vi "SV TDMS Read Even-Angle Channel Info.vi"(8 "error in":errorcluster, 9 "channel name in":string, 10 "group name in":string, 11 "tdms file":refnum<k34>) -> (0 "error out":errorcluster, 1 "channel name out":string, 2 "group name out":string, 3 "tdms file out":refnum<k34>, 4 "even-angle channel info":T2 {"channel info"."pregain" format="%.2f"; "channel info"."weighting filter" items=["Linear", "A-weighting", "B-weighting", "C-weighting", "ITU-R 468-4", "Dolby", "CCITT", "C-message", "Wb", "Wc", "Wd", "We", "Wf", "Wh", "Wj", "Wk", "Wm", "AES17 20 kHz lowpass", "AES17 40 kHz lowpass", "AES17 20 kHz highpass", "AES17 40 kHz highpass"]; "channel info"."dB reference" format="%^.1e"; "channel info"."engineering units" items=["custom..."=0, "V"=1, "A"=21, "C"=30, "pC"=31, "s"=32, "-"=29, "Pa"=2, "N"=20, "g"=3, "m/s^2"=4, "m/s"=5, "m"=6, "mm/s"=12, "mm"=13, "micron/s"=14, "micron"=15, "in/s^2"=7, "in/s"=8, "in"=9, "mil/s"=10, "mil"=11, "rad/s^2"=16, "rad/s"=17, "rad"=18, "deg/s^2"=26, "deg/s"=27, "deg"=28, "RPM"=22, "cycle/s^2"=23, "Hz"=24, "cycle"=25, "strain"=19]; "channel info"."sensor sensitivity" format="%#_5f"}, 6 "scale labels":T1)   [LabVIEW 2017]
uses:
  <vilib>/addons/_NISVFA/_Shared subVIs/Controls/svc_Resampled Channel Info.ctl
  <vilib>/addons/_NISVFA/_Shared subVIs/Controls/svc_Channel Info.ctl
  <vilib>/addons/_NISVFA/_Shared subVIs/Controls/svc_Engineering Units Text Ring.ctl
  <vilib>/addons/_NISVFA/_Shared subVIs/Controls/svc_Weighting Filter Text Ring.ctl
  <vilib>/addons/_NISVFA/_Shared subVIs/Controls/NI Channel Properties.ctl
  <vilib>/addons/_NISVFA/_Shared subVIs/Controls/SV Channel Properties.ctl
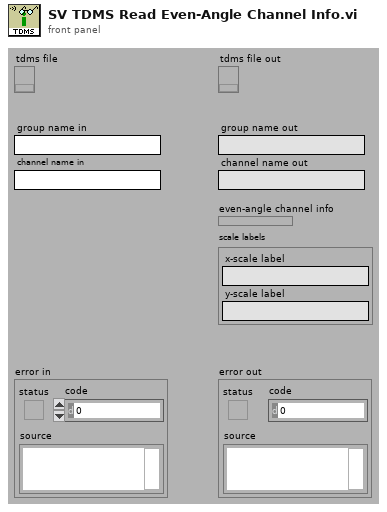
[diagram p1: front panel]
types:
  T1 = cluster{"x-scale label":string, "y-scale label":string}
  T2 = typedef "svc_Resampled Channel Info.ctl" = cluster{"channel name":string, "description":string, " channel info":T3}
  T3 = typedef "svc_Channel Info.ctl" = cluster{"sensor sensitivity":dbl, "engineering units":T4, "dB reference":dbl, "custom label":string, "weighting filter":T5, "pregain":dbl}
  T4 = typedef "svc_Engineering Units Text Ring.ctl" = u16
  T5 = typedef "svc_Weighting Filter Text Ring.ctl" = u16
  T6 = typedef "NI Channel Properties.ctl" = u16
  T7 = typedef "SV Channel Properties.ctl" = u16
  T8 = cluster{"scale label with units":string, "scale label with units":string}
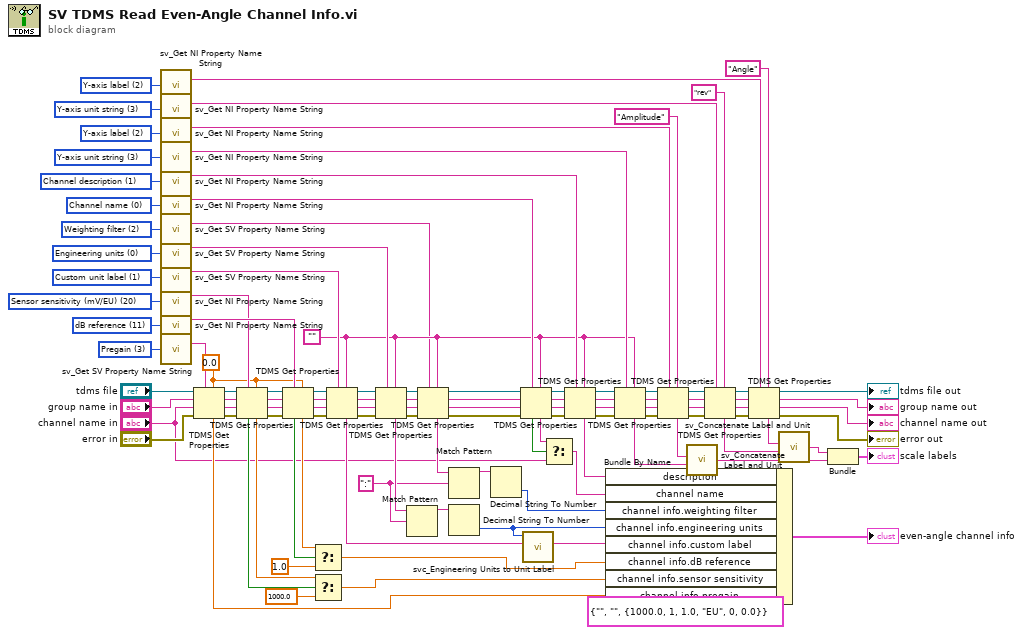
[diagram p0: block diagram]
diagram:
  w28 = T6 2 items=["Channel name", "Channel description", "Y-axis label", "Y-axis unit string", "X-axis label", "X-axis unit string", "x0", "dx", "Number of samples", "X channel", "Filter settled", "dB reference", "Window", "Window parameter", "Window size", "FFT size", "Peak units", "Spectrum type", "Magnitude scale", "Spectral density"] ("property")
  w27 = T6 3 items=["Channel name", "Channel description", "Y-axis label", "Y-axis unit string", "X-axis label", "X-axis unit string", "x0", "dx", "Number of samples", "X channel", "Filter settled", "dB reference", "Window", "Window parameter", "Window size", "FFT size", "Peak units", "Spectrum type", "Magnitude scale", "Spectral density"] ("property")
  w80 = T6 20 items=["Channel name", "Channel description", "Y-axis label", "Y-axis unit string", "X-axis label", "X-axis unit string", "x0", "dx", "Number of samples", "X channel", "Filter settled", "dB reference", "Window", "Window parameter", "Window size", "FFT size", "Peak units", "Spectrum type", "Magnitude scale", "Spectral density", "Sensor sensitivity (mV/EU)", "X-axis domain", "LabVIEW datatype"] ("property")
  w58 = ":" ("regular expression")
  w62 = "" ("channel info.custom label")
  w13 = 0.0 ("property values")
  w71 = T6 0 items=["Channel name", "Channel description", "Y-axis label", "Y-axis unit string", "X-axis label", "X-axis unit string", "x0", "dx", "Number of samples", "X channel", "Filter settled", "dB reference", "Window", "Window parameter", "Window size", "FFT size", "Peak units", "Spectrum type", "Magnitude scale", "Spectral density", "Sensor sensitivity (mV/EU)"] ("property")
  w74 = T6 11 items=["Channel name", "Channel description", "Y-axis label", "Y-axis unit string", "X-axis label", "X-axis unit string", "x0", "dx", "Number of samples", "X channel", "Filter settled", "dB reference", "Window", "Window parameter", "Window size", "FFT size", "Peak units", "Spectrum type", "Magnitude scale", "Spectral density"] ("property")
  w75 = T7 3 items=["Engineering units", "Custom unit label", "Weighting filter", "Pregain", "Octave standard", "Octave bandwidth", "Octave low band", "Octave high band", "Spectrum skewed"] ("SV property")
  w79 = T6 2 items=["Channel name", "Channel description", "Y-axis label", "Y-axis unit string", "X-axis label", "X-axis unit string", "x0", "dx", "Number of samples", "X channel", "Filter settled", "dB reference", "Window", "Window parameter", "Window size", "FFT size", "Peak units", "Spectrum type", "Magnitude scale", "Spectral density"] ("property")
  w81 = T7 1 items=["Engineering units", "Custom unit label", "Weighting filter", "Pregain", "Octave standard", "Octave bandwidth", "Octave low band", "Octave high band", "Spectrum skewed"] ("SV property")
  w82 = T7 0 items=["Engineering units", "Custom unit label", "Weighting filter", "Pregain", "Octave standard", "Octave bandwidth", "Octave low band", "Octave high band", "Spectrum skewed"] ("SV property")
  w84 = T7 2 items=["Engineering units", "Custom unit label", "Weighting filter", "Pregain", "Octave standard", "Octave bandwidth", "Octave low band", "Octave high band", "Spectrum skewed"] ("SV property")
  w85 = T6 1 items=["Channel name", "Channel description", "Y-axis label", "Y-axis unit string", "X-axis label", "X-axis unit string", "x0", "dx", "Number of samples", "X channel", "Filter settled", "dB reference", "Window", "Window parameter", "Window size", "FFT size", "Peak units", "Spectrum type", "Magnitude scale", "Spectral density"] ("property")
  w83 = T6 3 items=["Channel name", "Channel description", "Y-axis label", "Y-axis unit string", "X-axis label", "X-axis unit string", "x0", "dx", "Number of samples", "X channel", "Filter settled", "dB reference", "Window", "Window parameter", "Window size", "FFT size", "Peak units", "Spectrum type", "Magnitude scale", "Spectral density"] ("property")
  n1 = call <vilib>:"sv_Get NI Property Name String.vi"("property"=w28) -> ("TDMS property name"=w25:string)  [unwired: 13 in, 1 out]
  n2 = call <vilib>:"sv_Get NI Property Name String.vi"("property"=w27) -> ("TDMS property name"=w26:string)  [unwired: 13 in, 1 out]
  n3 = call <vilib>:"sv_Get NI Property Name String.vi"("property"=w79) -> ("TDMS property name"=w65:string)  [unwired: 13 in, 1 out]
  n4 = call <vilib>:"sv_Get NI Property Name String.vi"("property"=w83) -> ("TDMS property name"=w78:string)  [unwired: 13 in, 1 out]
  n5 = call <vilib>:"sv_Get NI Property Name String.vi"("property"=w85) -> ("TDMS property name"=w77:string)  [unwired: 13 in, 1 out]
  n6 = call <vilib>:"sv_Get NI Property Name String.vi"("property"=w71) -> ("TDMS property name"=w70:string)  [unwired: 13 in, 1 out]
  n7 = call <vilib>:"sv_Get SV Property Name String.vi"("property"=w84) -> ("TDMS property name"=w61:string)  [unwired: 13 in, 1 out]
  n8 = call <vilib>:"sv_Get SV Property Name String.vi"("property"=w82) -> ("TDMS property name"=w64:string)  [unwired: 13 in, 1 out]
  n9 = call <vilib>:"sv_Get SV Property Name String.vi"("property"=w81) -> ("TDMS property name"=w76:string)  [unwired: 13 in, 1 out]
  n10 = call <vilib>:"sv_Get NI Property Name String.vi"("property"=w80) -> ("TDMS property name"=w60:string)  [unwired: 13 in, 1 out]
  n11 = call <vilib>:"sv_Get NI Property Name String.vi"("property"=w74) -> ("TDMS property name"=w72:string)  [unwired: 13 in, 1 out]
  n12 = call <vilib>:"sv_Get SV Property Name String.vi"("property"=w75) -> ("TDMS property name"=w73:string)  [unwired: 13 in, 1 out]
  n13 = TDMS Get Properties(5:w13, 7:w73, 8:"error in", 9:"channel name in", 10:"group name in", 11:"tdms file") -> (0:w53:errorcluster, 1:w54:string, 2:w55:string, 3:w56:refnum<k34>, 4:w5:dbl)  [unwired: 1 out]
  n14 = TDMS Get Properties(5:w13, 7:w60, 8:w53, 9:w54, 10:w55, 11:w56) -> (0:w52:errorcluster, 1:w51:string, 2:w50:string, 3:w49:refnum<k34>, 4:w9:dbl, 6:w7:bool)
  n15 = TDMS Get Properties(5:w13, 7:w72, 8:w52, 9:w51, 10:w50, 11:w49) -> (0:w86:errorcluster, 1:w87:string, 2:w88:string, 3:w89:refnum<k34>, 4:w11:dbl, 6:w14:bool)
  n16 = Select(t=w11, s=w14, f=1.0) -> (s? t:f=w10:dbl)
  n17 = Select(t=w9, s=w7, f=1000.0) -> (s? t:f=w8:dbl)
  n18 = TDMS Get Properties(5:w62, 7:w76, 8:w86, 9:w87, 10:w88, 11:w89) -> (0:w112:errorcluster, 1:w111:string, 2:w110:string, 3:w109:refnum<k34>, 4:w17:string)  [unwired: 1 out]
  n19 = TDMS Get Properties(5:w62, 7:w64, 8:w112, 9:w111, 10:w110, 11:w109) -> (0:w105:errorcluster, 1:w106:string, 2:w107:string, 3:w108:refnum<k34>, 4:w63:string)  [unwired: 1 out]
  n20 = Match Pattern(string=w63, regular expression=w58) -> (before substring=w69:string)  [unwired: 1 in, 3 out]
  n21 = TDMS Get Properties(5:w62, 7:w61, 8:w105, 9:w106, 10:w107, 11:w108) -> (0:w48:errorcluster, 1:w47:string, 2:w46:string, 3:w45:refnum<k34>, 4:w59:string)  [unwired: 1 out]
  n22 = Match Pattern(string=w59, regular expression=w58) -> (before substring=w67:string)  [unwired: 1 in, 3 out]
  n23 = Decimal String To Number(string=w69) -> (number=w15:i32)  [unwired: 2 in, 1 out]
  n24 = Decimal String To Number(string=w67) -> (number=w57:i32)  [unwired: 2 in, 1 out]
  n25 = TDMS Get Properties(5:w62, 7:w70, 8:w48, 9:w47, 10:w46, 11:w45) -> (0:w104:errorcluster, 1:w103:string, 2:w102:string, 3:w101:refnum<k34>, 4:w2:string, 6:w4:bool)
  n26 = call <vilib>:"svc_Engineering Units to Unit Label.vi"("custom label"=w17, "engineering units"=w15) -> ("unit label"=w16:string)  [unwired: 8 in, 1 out]
  n27 = Select(t=w2, s=w4, f="channel name in") -> (s? t:f=w1:string)
  n28 = TDMS Get Properties(5:w62, 7:w77, 8:w104, 9:w103, 10:w102, 11:w101) -> (0:w90:errorcluster, 1:w91:string, 2:w92:string, 3:w93:refnum<k34>, 4:w44:string)  [unwired: 1 out]
  n29 = Bundle By Name(cluster=T2 {"channel name"="", "description"="", " channel info"={"sensor sensitivity"=1000.0, "engineering units"=1, "dB reference"=1.0, "custom label"="EU", "weighting filter"=0, "pregain"=0.0}} ("input cluster"), "description"=w44, "channel name"=w1, "channel info.weighting filter"=w57, "channel info.engineering units"=w15, "channel info.custom label"=w16, "channel info.dB reference"=w10, "channel info.sensor sensitivity"=w8, "channel info.pregain"=w5) -> (→"even-angle channel info":T2)
  n30 = TDMS Get Properties(5:w62, 7:w78, 8:w90, 9:w91, 10:w92, 11:w93) -> (0:w97:errorcluster, 1:w96:string, 2:w95:string, 3:w94:refnum<k34>, 4:w42:string)  [unwired: 1 out]
  n31 = TDMS Get Properties(5:"Amplitude" ("channel name"), 7:w65, 8:w97, 9:w96, 10:w95, 11:w94) -> (0:w40:errorcluster, 1:w39:string, 2:w38:string, 3:w37:refnum<k34>, 4:w43:string)  [unwired: 1 out]
  n32 = call <vilib>:"sv_Concatenate Label and Unit.vi"("unit string"=w42, "label"=w43) -> ("scale label with units"=w41:string)  [unwired: 4 in]
  n33 = TDMS Get Properties(5:"rev" ("channel name"), 7:w26, 8:w40, 9:w39, 10:w38, 11:w37) -> (0:w36:errorcluster, 1:w35:string, 2:w34:string, 3:w33:refnum<k34>, 4:w21:string)  [unwired: 1 out]
  n34 = TDMS Get Properties(5:"Angle" ("channel name"), 7:w25, 8:w36, 9:w35, 10:w34, 11:w33) -> (0:→"error out":errorcluster, 1:→"channel name out":string, 2:→"group name out":string, 3:→"tdms file out":refnum<k34>, 4:w22:string)  [unwired: 1 out]
  n35 = call <vilib>:"sv_Concatenate Label and Unit.vi"("unit string"=w21, "label"=w22) -> ("scale label with units"=w20:string)  [unwired: 4 in]
  n36 = Bundle("scale label with units"=w20, "scale label with units"=w41) -> (→"scale labels":T8)  [unwired: 1 in]
